vi "Write One-Second Interval Message.vi"(8 "Error In":errorcluster, 11 "Unhandled Errors":T1[](array[typedef])) -> (0 "Error Out":errorcluster)   [LabVIEW 2023, in "Error Manager.lvlib"]
uses:
  Error Manager.lvlib
  Unhandled Error (cluster).ctl
  Error Log/Error Log.lvclass
panel:
  out "Text written to log":string
  # "Input\nInputs to the VI"
  # "Development\nControls or indicators that are useful for development or testing, but which are not outputs of the VI."
  # "Output\nOutputs of the VI"
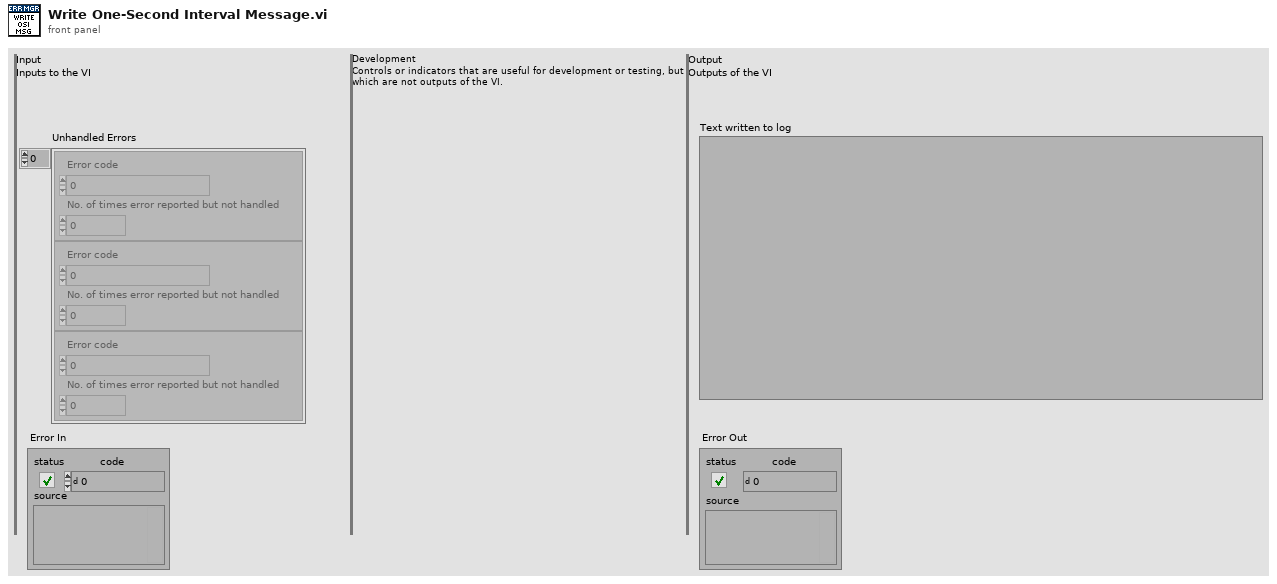
[diagram p1: front panel]
types:
  T1 = typedef "Error Manager.lvlib/Unhandled Error (cluster).ctl" = cluster{"Error code":i32, "No. of times error reported but not handled":u32}
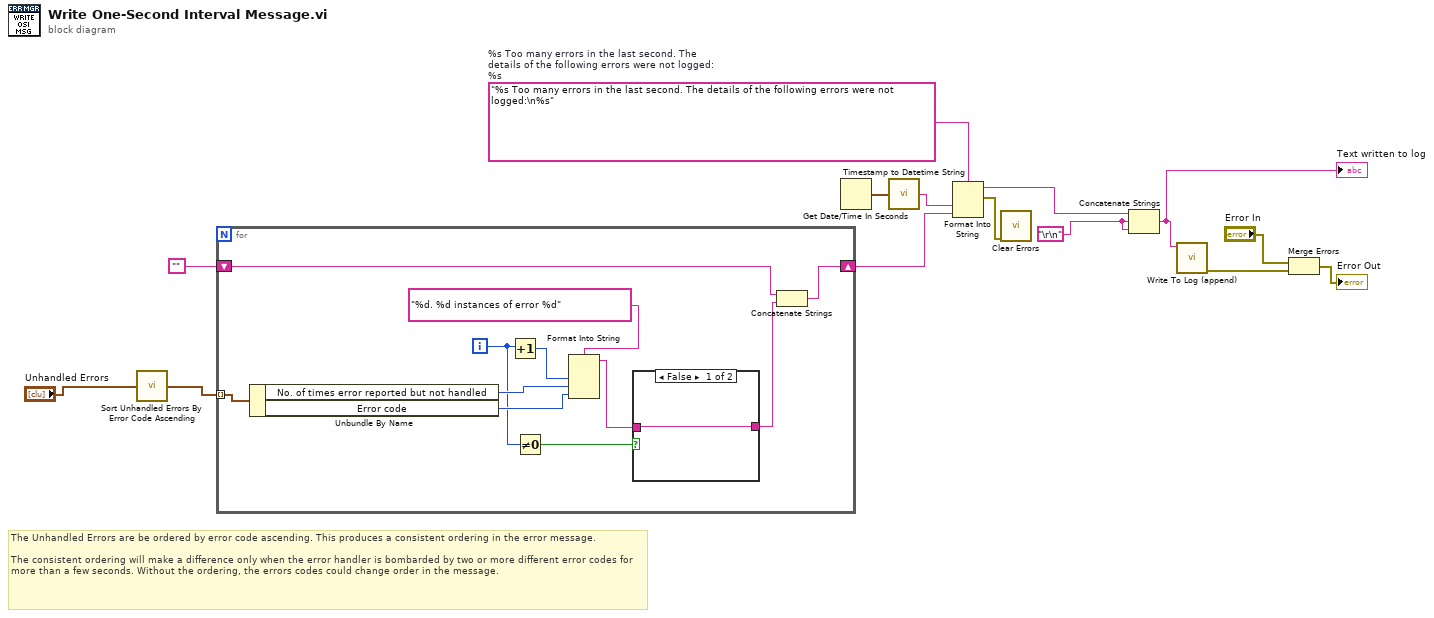
[diagram p0: block diagram]
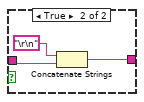
[diagram p2: hidden frame]
diagram:
  w7 = "\r\n"
  w11 = "%s Too many errors in the last second. The details of the following errors were not logged:\n%s"  # %s Too many errors in the last second. The details of the following errors were not logged: %s
  # "The Unhandled Errors are be ordered by error code ascending. This produces a consistent ordering in the error message. \n\nThe consistent ordering will make a difference only when the error handler is bombarded by two or more different error codes for more than a few seconds. Without the ordering, the errors codes could change order in the message."
  n1 = call "Sort Unhandled Errors By Error Code Ascending.vi"("Unhandled Errors (unsorted)"="Unhandled Errors") -> ("Unhandled Errors (sorted by error code, ascending)"=w1:T1[])
  n2 = for {
    tunnel: w1 -> [w23] mode=indexing
    shift-right: [w16] -> w3
    shift-left: "" -> [w17]
    i -> [w20]
    n3 = Unbundle By Name(w23) -> ("No. of times error reported but not handled"=w22:u32, "Error code"=w21:i32)
    n4 = Increment(x=w20) -> (x+1=w25:i32)
    n5 = Not Equal To 0?(x=w20) -> (x != 0?=w19:bool)
    n6 = Format Into String(format string="%d. %d instances of error %d", w25, w22, w21) -> (resulting string=w18:string)  [unwired: 2 in, 1 out]
    n7 = case shown="False" w19 {
      tunnel: w18 -> [w26 w29]
      tunnel: [w26 w27] -> w15
      frame False {
      }
      frame True {
        n8 = Concatenate Strings("\r\n", w29) -> (w27:string)
      }
    }
    n9 = Concatenate Strings(w17, w15) -> (w16:string)
  }
  n10 = Get Date/Time In Seconds() -> (seconds since 1Jan1904=w6:timestamp)
  n11 = call "Timestamp to Datetime String.vi"("Timestamp"=w6) -> ("Date-Time String"=w5:string)
  n12 = Format Into String(format string=w11, w5, w3) -> (resulting string=w10:string, error out=w8:errorcluster)  [unwired: 2 in]
  n13 = call <vilib>:"Clear Errors.vi"("error in (no error)"=w8) -> ()  [unwired: 5 in, 2 out]
  n14 = Concatenate Strings(w10, w7, w7) -> (w9:string)
  "Text written to log" <- w9
  n15 = call "Write To Log (append).vi"("Text to write"=w9) -> ("error out"=w12:errorcluster)  [unwired: 10 in]
  n16 = Merge Errors("Error In", w12) -> (→"Error Out":errorcluster)
